vi "csvtest.vi"   [LabVIEW 2013]
uses:
  <vilib>/Utility/file.llb/Write To Spreadsheet File (I64).vi
  <vilib>/Utility/file.llb/Write To Spreadsheet File (DBL).vi
  <vilib>/Utility/file.llb/Write To Spreadsheet File (string).vi
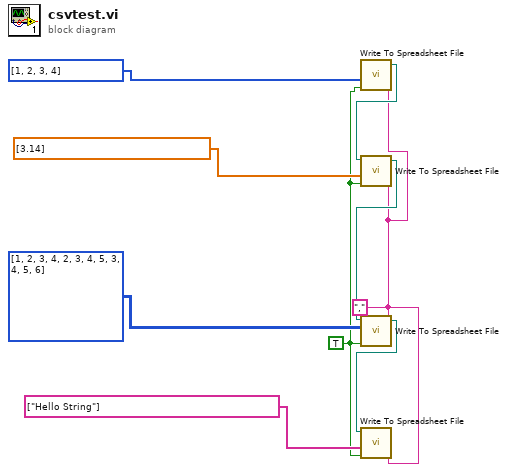
[diagram p0: block diagram]
diagram:
  w2 = "," ("delimiter (\\t)")
  w1 = TRUE ("append to file? (new file:F)")
  n1 = call-poly <vilib>:"Write To Spreadsheet File.vi"("delimiter (\\t)"=w2, "append to file? (new file:F)"=w1, "1D data"=i32[] [1, 2, 3, 4]) -> ("new file path (Not A Path if cancelled)"=w6:path)  [unwired: 5 in]
  n2 = call-poly <vilib>:"Write To Spreadsheet File.vi"("delimiter (\\t)"=w2, "append to file? (new file:F)"=w1, "1D data"=dbl[] [3.14], "file path (dialog if empty)"=w6) -> ("new file path (Not A Path if cancelled)"=w5:path)  [unwired: 4 in]
  n3 = call-poly <vilib>:"Write To Spreadsheet File.vi"("delimiter (\\t)"=w2, "append to file? (new file:F)"=w1, "2D data"=i32[][] [[1, 2, 3, 4], [2, 3, 4, 5], [3, 4, 5, 6]], "file path (dialog if empty)"=w5) -> ("new file path (Not A Path if cancelled)"=w3:path)  [unwired: 4 in]
  n4 = call-poly <vilib>:"Write To Spreadsheet File.vi"("delimiter (\\t)"=w2, "append to file? (new file:F)"=w1, "1D data"=string[] ["Hello String"], "file path (dialog if empty)"=w3) -> ()  [unwired: 4 in, 1 out]
